vi "fgv_gridmap_config.vi"(7 "cmd":T3, 11 "pf-val":T2={"xy_resolution"=0.0, "EXTEND_AREA"=0.0, "MAX_RANGE"=0.0, "NP"=0, "NTh"=0, "Q"=[[0.04000000000000001]], "R"=[[4.0, 0.0], [0.0, 0.4873878716587337]], "Q_sim"=[[0.04000000000000001]], "R_sim"=[[1.0, 0.0], [0.0, 0.2741556778080377]], "rf_id"=[{"x"=10.0, "y"=0.0}, {"x"=10.0, "y"=10.0}, {"x"=0.0, "y"=15.0}, {"x"=-5.0, "y"=20.0}], "map x size"=0, "map y size"=0, "map x center"=0, "map y center"=0}) -> (3 "pf-val out":T2={"xy_resolution"=0.0, "EXTEND_AREA"=0.0, "MAX_RANGE"=0.0, "NP"=0, "NTh"=0, "Q"=[[0.04000000000000001]], "R"=[[4.0, 0.0], [0.0, 0.4873878716587337]], "Q_sim"=[[0.04000000000000001]], "R_sim"=[[1.0, 0.0], [0.0, 0.2741556778080377]], "rf_id"=[{"x"=10.0, "y"=0.0}, {"x"=10.0, "y"=10.0}, {"x"=0.0, "y"=15.0}, {"x"=-5.0, "y"=20.0}], "map x size"=0, "map y size"=0, "map x center"=0, "map y center"=0})   [LabVIEW 2019]
uses:
  Ctrl/cmd_common.ctl
  <vilib>/Analysis/Matrix/Datatypes/RealMatrix.ctl
  <vilib>/Analysis/Matrix/NI_Matrix.lvlib
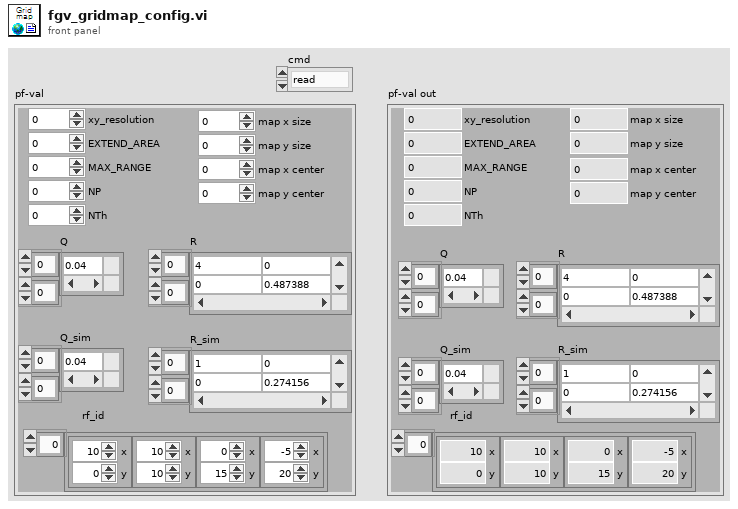
[diagram p1: front panel]
types:
  T1 = typedef "NI_Matrix.lvlib/RealMatrix.ctl" = dbl[][]
  T2 = cluster{"xy_resolution":dbl, "EXTEND_AREA":dbl, "MAX_RANGE":dbl, "NP":u32, "NTh":u32, "Q":T1, "R":T1, "Q_sim":T1, "R_sim":T1, "rf_id":cluster{"x":dbl, "y":dbl}[], "map x size":u32, "map y size":u32, "map x center":u32, "map y center":u32}
  T3 = typedef "cmd_common.ctl" = enum16{"read", "write"}
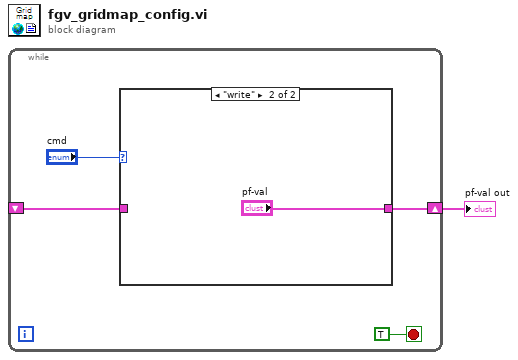
[diagram p0: block diagram]
diagram:
  n1 = while {
    shift-right: [w3] -> w1
    shift-left: _ -> [w2]
    stop <- TRUE stop-if-true
    n2 = case shown="\"write\"" "cmd" {
      tunnel: [w6 "pf-val"] -> w3
      tunnel: w2 -> [w6 _]
      frame "read", Default {
      }
      frame "write" {
      }
    }
  }
  "pf-val out" <- w1
